vi "dfd_ZPK to SOS.vi"(8 "UP?":bool, 9 "gain":dbl=1.0, 10 "poles":cdb[](array[numeric]), 11 "zeros":cdb[](array[numeric])) -> (2 "SOS reverse coefficients":dbl[](array[numeric]), 3 "SOS forward coefficients":dbl[](array[numeric]))   [LabVIEW 2017, in "NI_DigFilterLicensed.lvlib"]
uses:
  <vilib>/addons/Digital Filter Design/NI_DigFilterLicensed.lvlib
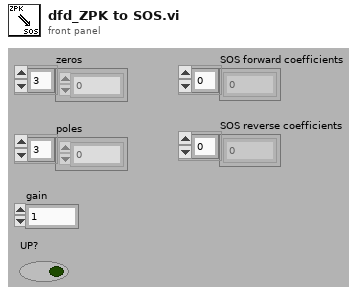
[diagram p1: front panel]
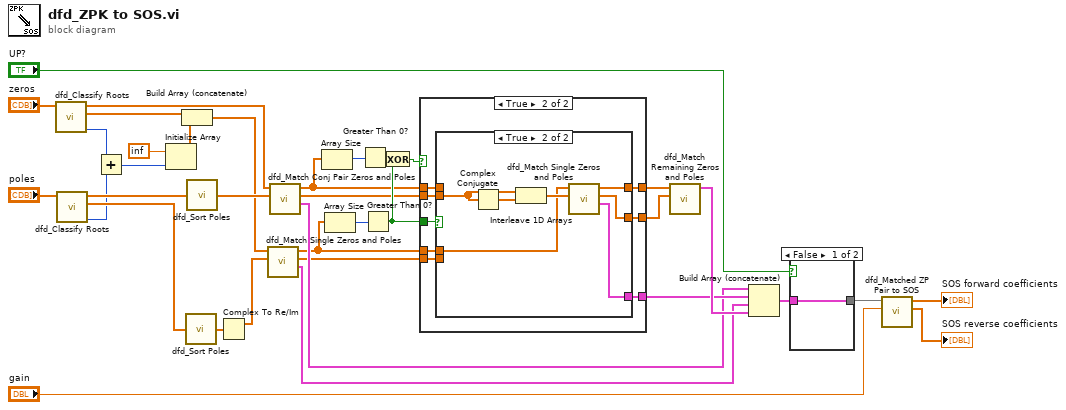
[diagram p0: block diagram]
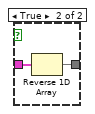
[diagram p2: hidden frame]
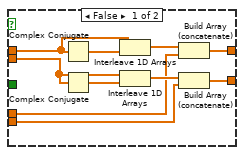
[diagram p3: hidden frame]
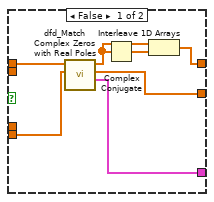
[diagram p4: hidden frame]
diagram:
  n1 = call <vilib>:"dfd_Classify Roots.vi"("Roots"="zeros") -> ("# zero-inf root"=w2:i32, "real roots"=w12:dbl[], "conj roots"=w31:cdb[])  [unwired: 8 out]
  n2 = call <vilib>:"dfd_Classify Roots.vi"("Roots"="poles") -> ("# zero-inf root"=w3:i32, "real roots"=w36:dbl[], "conj roots"=w35:cdb[])  [unwired: 8 out]
  n3 = Add(x=w2, y=w3) -> (x+y=w7:i32)
  n4 = Initialize Array(inf, w7) -> (w9:dbl[])
  n5 = Build Array (concatenate)(w12, w9) -> (w10:dbl[])
  n6 = call <vilib>:"dfd_Sort Poles.vi"("poles"=w36) -> ("sorted poles"=w13:cdb[])
  n7 = call <vilib>:"dfd_Sort Poles.vi"("poles"=w35) -> ("sorted poles"=w32:cdb[])
  n8 = Complex To Re/Im(x + iy=w13) -> (x=w14:dbl[])  [unwired: 1 out]
  n9 = call <vilib>:"dfd_Match Single Zeros and Poles.vi"("real poles"=w14, "real zeros"=w10) -> ("matched z&p"=w1:cluster{"zeros":cdb[], "poles":cdb[]}[], "remaining poles"=w19:cdb[], "remaining zeros"=w18:cdb[])  [unwired: 7 out]
  n10 = call <vilib>:"dfd_Match Conj Pair Zeros and Poles.vi"("conj poles"=w32, "conj zeros"=w31) -> ("matched z&p"=w26:cluster{"zeros":cdb[], "poles":cdb[]}[], "remaining poles"=w20:cdb[], "remaining zeros"=w17:cdb[])  [unwired: 7 out]
  n11 = Array Size(array=w17) -> (size(s)=w15:i32)
  n12 = Array Size(array=w18) -> (size(s)=w16:i32)
  n13 = Greater Than 0?(x=w15) -> (x > 0?=w21:bool)
  n14 = Greater Than 0?(x=w16) -> (x > 0?=w22:bool)
  n15 = Exclusive Or(1:w22, 2:w21) -> (0:w23:bool)
  n16 = case shown="True" w23 {
    tunnel: w22 -> [_ w54]
    tunnel: w17 -> [w42 w53]
    tunnel: w18 -> [w40 w52]
    tunnel: w19 -> [w39 w51]
    tunnel: [w38 w49] -> w24
    tunnel: w20 -> [w41 w50]
    tunnel: [w37 w48] -> w25
    tunnel: [_ w47] -> w27
    frame False {
      n17 = Complex Conjugate(1:w42) -> (0:w46:cdb[])
      n18 = Complex Conjugate(1:w41) -> (0:w45:cdb[])
      n19 = Interleave 1D Arrays(w42, w46) -> (w44:cdb[])
      n20 = Interleave 1D Arrays(w41, w45) -> (w43:cdb[])
      n21 = Build Array (concatenate)(w44, w40) -> (w38:cdb[])
      n22 = Build Array (concatenate)(w43, w39) -> (w37:cdb[])
    }
    frame True {
      n23 = case shown="True" w54 {
        tunnel: w53 -> [w59 _]
        tunnel: w52 -> [_ w65]
        tunnel: w51 -> [w61 _]
        tunnel: w50 -> [_ w67]
        tunnel: [w55 w64] -> w49
        tunnel: [w60 w62] -> w48
        tunnel: [w58 w63] -> w47
        frame False {
          n24 = call <vilib>:"dfd_Match Complex Zeros with Real Poles.vi"("real poles"=w61, "conj zeros"=w59) -> ("matched z&p"=w58:cluster{"zeros":cdb[], "poles":cdb[]}[], "remaining poles"=w60:cdb[], "remaining zeros"=w56:cdb[])  [unwired: 7 out]
          n25 = Complex Conjugate(1:w56) -> (0:w57:cdb[])
          n26 = Interleave 1D Arrays(w56, w57) -> (w55:cdb[])
        }
        frame True {
          n27 = Complex Conjugate(1:w67) -> (0:w68:cdb[])
          n28 = Interleave 1D Arrays(w67, w68) -> (w66:cdb[])
          n29 = call <vilib>:"dfd_Match Single Zeros and Poles.vi"("real poles"=w66, "real zeros"=w65) -> ("matched z&p"=w63:cluster{"zeros":cdb[], "poles":cdb[]}[], "remaining poles"=w62:cdb[], "remaining zeros"=w64:cdb[])  [unwired: 7 out]
        }
      }
    }
  }
  n30 = call <vilib>:"dfd_Match Remaining Zeros and Poles.vi"("remaining poles"=w25, "remaining zeros"=w24) -> ("matched zeros and poles"=w28:cluster{cdb[], cdb[]}[])  [unwired: 9 out]
  n31 = Build Array (concatenate)(w26, w27, w1, w28) -> (w6:cluster{"zeros":cdb[], "poles":cdb[]}[])
  n32 = case shown="False" "UP?" {
    tunnel: w6 -> [w69 w71]
    tunnel: [w69 w70] -> w4
    frame False {
    }
    frame True {
      n33 = Reverse 1D Array(array=w71) -> (reversed array=w70:cluster{"zeros":cdb[], "poles":cdb[]}[])
    }
  }
  n34 = call <vilib>:"dfd_Matched ZP Pair to SOS.vi"("gain"="gain", "Matched ZP Pair"=w4) -> ("SOS reverse coefficients"=→"SOS reverse coefficients":dbl[], "SOS forward coefficients"=→"SOS forward coefficients":dbl[])  [unwired: 8 out]
